vi "PS Ref.vi"(7 "CMD":T1, 8 "error in (no error)":errorcluster, 11 "PalmSens.lvclass":refnum<class "PalmSens.lvclass">) -> (0 "error out":errorcluster, 3 "PalmSens.lvclass out":refnum<class "PalmSens.lvclass">)   [LabVIEW 2020]
uses:
  <instrlib>/PalmSens SDK for LabVIEW 5.10/PalmSens/PalmSens.lvclass
  PCT FGV CMD.ctl
panel:
  in  "PalmSens.lvclass 2":refnum<class "PalmSens.lvclass">
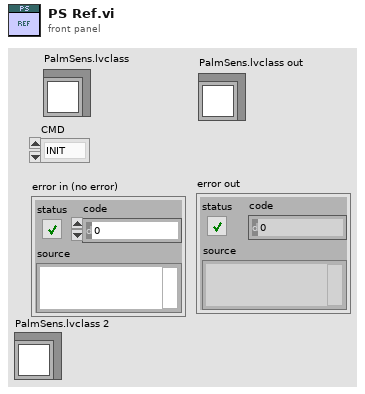
[diagram p1: front panel]
types:
  T1 = typedef "PCT FGV CMD.ctl" = enum16{"INIT", "GET", "SET"}
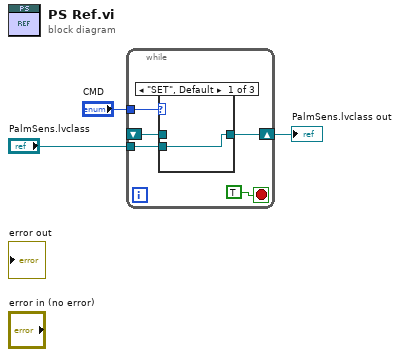
[diagram p0: block diagram]
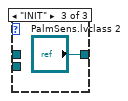
[diagram p3: hidden frame]
diagram:
  n1 = while {
    tunnel: "PalmSens.lvclass" -> [w6]
    tunnel: "CMD" -> [w8]
    shift-right: [w5] -> w3
    shift-left: _ -> [w7]
    stop <- TRUE stop-if-true
    n2 = case shown="\"SET\", Default" w8 {
      tunnel: w7 -> [_ w10 _]
      tunnel: w6 -> [w9 _ _]
      tunnel: [w9 w10 "PalmSens.lvclass 2"] -> w5
      frame "SET", Default {
      }
      frame "GET" {
      }
      frame "INIT" {
      }
    }
  }
  "PalmSens.lvclass out" <- w3
